vi "Reader Object Reference..FGV.vi"(6 "Connection Name":string, 7 "FGV State (GET)":T1, 8 "error in (no error)":errorcluster, 11 "Reader ref in":refnum<k24>) -> (0 "error out":errorcluster, 3 "Reader ref out":refnum<k24>)   [LabVIEW 2015, in "LabSSH.lvlib"]
doc: "<License>This software is distributed under the BSD 3-Clause License. For the full license please see license.txt or visit www.labvolution.com/license</License>"
uses:
  LabSSH.lvlib
  FGV State..enum.ctl
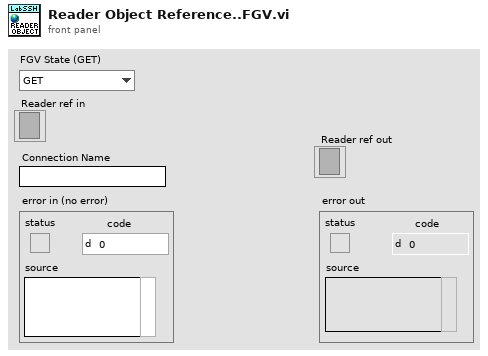
[diagram p1: front panel]
types:
  T1 = typedef "LabSSH.lvlib/FGV State..enum.ctl" = enum16{"GET", "SET"}
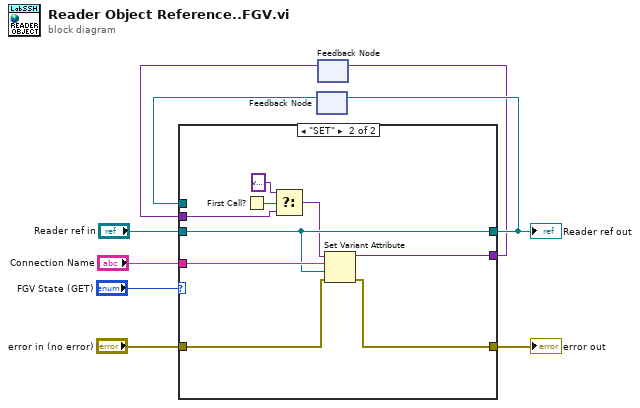
[diagram p0: block diagram]
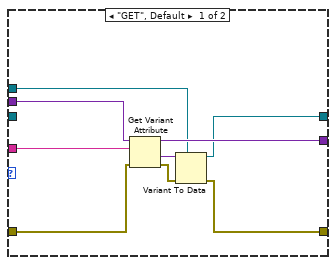
[diagram p2: hidden frame]
diagram:
  n1 = feedback #1() -> (w6:refnum<k24>)  [unwired: 1 in]
  n2 = feedback #2() -> (w1:variant)  [unwired: 1 in]
  n3 = case shown="\"SET\"" "FGV State (GET)" {
    tunnel: "error in (no error)" -> [w15 w25]
    tunnel: [w14 w24] -> w8
    tunnel: "Reader ref in" -> [_ w26]
    tunnel: [w11 w26] -> w4
    tunnel: w6 -> [w12 _]
    tunnel: "Connection Name" -> [w13 w27]
    tunnel: [w16 w23] -> w2
    tunnel: w1 -> [w10 w20]
    frame "GET", Default {
      n4 = Get Variant Attribute(Variant=w10, name=w13, error in=w15) -> (duplicate Variant=w16:variant, value=w17:variant, error out=w18:errorcluster)  [unwired: 1 in, 1 out]
      n5 = Variant To Data(error in=w18, type=w12, Variant=w17) -> (data=w11:refnum<k24>, error out=w14:errorcluster)
    }
    frame "SET" {
      n6 = First Call?() -> (First Call?: T/F=w21:bool)
      n7 = Select(t=variant ("variant"), s=w21, f=w20) -> (s? t:f=w19:variant)
      n8 = Set Variant Attribute(Variant=w19, name=w27, value=w26, error in=w25) -> (Variant out=w23:variant, error out=w24:errorcluster)  [unwired: 1 out]
    }
  }
  "error out" <- w8
  "Reader ref out" <- w4
  n9 = feedback-in #1(w4) -> ()
  n10 = feedback-in #2(w2) -> ()
